vi "libdaq_dac_stop.vi"(0 "error in (no error)":errorcluster, 1 "device_name":string, 2 "module_name":string) -> (14 "error out":errorcluster, 15 "device_name":string, 16 "module_name":string)   [LabVIEW 2010, in "libdaqVI.lvlib"]
doc: "停止DAC模块的输出，对所有触发模式有效；当为硬件触发模式(HARD)时，通过该函数停止DAC模块输出后，无法通过libdaq_dac_start函数触发输出，只能再次等待硬件触发。该命令起作用后DAC将会保持最后一次的输出结果。"
uses:
  libdaqVI.lvlib
  dll/daqlib.dll
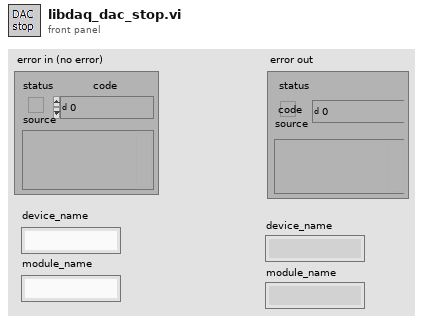
[diagram p1: front panel]
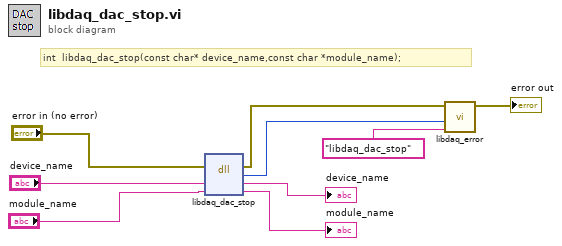
[diagram p0: block diagram]
diagram:
  # "int  libdaq_dac_stop(const char* device_name,const char *module_name);"
  n1 = dll-call lib="E:/Product/Example/DAQ-USB3212/Labview/labview_2010/libdaqVI/dll/daqlib.dll" fn="libdaq_dac_stop"(error in="error in (no error)", "device_name"="device_name", "module_name"="module_name") -> (error out=w2:errorcluster, "return type"=w4:i32, "device_name"=→"device_name":string, "module_name"=→"module_name":string)  [unwired: 2 in, 1 out]
  n2 = call "libdaq_error.vi"("error source"="libdaq_dac_stop", "error code"=w4, "错误输入（无错误）"=w2) -> ("错误输出"=→"error out":errorcluster)  [unwired: 8 in]
